vi "ArrayBuffer_main.vi"() -> ()   [LabVIEW 2020]
uses:
  <vilib>/numeric/Random Number (Range) U64.vi
  <vilib>/numeric/sub_Random U32.vi
  Desktop/AddrToValue.dll
  Desktop/Dll_Lib_DAQ_Child.dll
  Desktop/Dll_Lib_DAQ.dll
panel:
  out "First Run Com?":bool
  out "initialized array 2":i32[](array[numeric])
  out "initialized array":i32[](array[numeric])
  out "DBL 2":dbl
  out "string 2":string
  out "Array":i32[](array[numeric])
  out "string":string
  out "error out":errorcluster
  out "DBL":dbl
  in  "input":T1={"DBL"=10.0, "String (50 Character Limit)"="abcd", "Array (50 Element Limit)"=[10, 100]}
  out "output array":i32[](array[numeric])
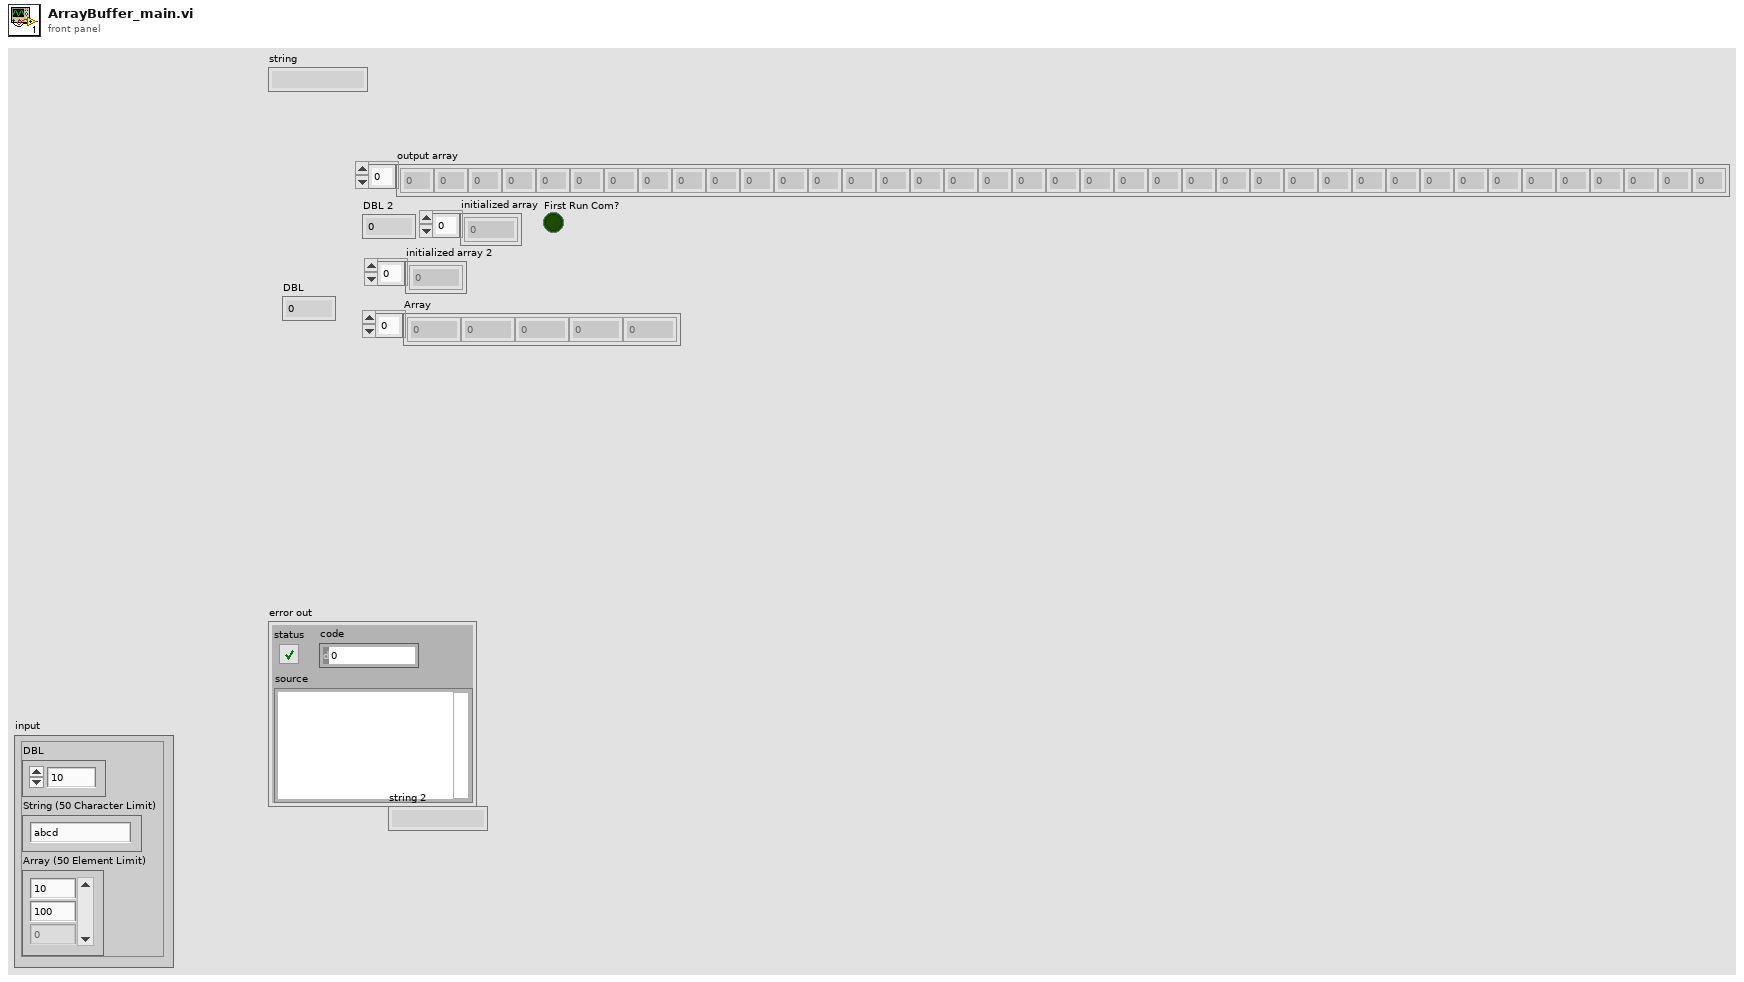
[diagram p1: front panel]
types:
  T1 = cluster{"DBL":dbl, "String (50 Character Limit)":string, "Array (50 Element Limit)":i32[]}
  T2 = cluster{"unsigned byte array[0]":u8, "unsigned byte array[1]":u8, "unsigned byte array[2]":u8, "unsigned byte array[3]":u8, "unsigned byte array[4]":u8, "unsigned byte array[5]":u8, "unsigned byte array[6]":u8, "unsigned byte array[7]":u8, "unsigned byte array[8]":u8, "unsigned byte array[9]":u8, "unsigned byte array[10]":u8, "unsigned byte array[11]":u8, "unsigned byte array[12]":u8, "unsigned byte array[13]":u8, "unsigned byte array[14]":u8, "unsigned byte array[15]":u8, "unsigned byte array[16]":u8, "unsigned byte array[17]":u8, "unsigned byte array[18]":u8, "unsigned byte array[19]":u8, "unsigned byte array[20]":u8, "unsigned byte array[21]":u8, "unsigned byte array[22]":u8, "unsigned byte array[23]":u8, "unsigned byte array[24]":u8, "unsigned byte array[25]":u8, "unsigned byte array[26]":u8, "unsigned byte array[27]":u8, "unsigned byte array[28]":u8, "unsigned byte array[29]":u8, "unsigned byte array[30]":u8, "unsigned byte array[31]":u8, "unsigned byte array[32]":u8, "unsigned byte array[33]":u8, "unsigned byte array[34]":u8, "unsigned byte array[35]":u8, "unsigned byte array[36]":u8, "unsigned byte array[37]":u8, "unsigned byte array[38]":u8, "unsigned byte array[39]":u8, "unsigned byte array[40]":u8, "unsigned byte array[41]":u8, "unsigned byte array[42]":u8, "unsigned byte array[43]":u8, "unsigned byte array[44]":u8, "unsigned byte array[45]":u8, "unsigned byte array[46]":u8, "unsigned byte array[47]":u8, "unsigned byte array[48]":u8, "unsigned byte array[49]":u8, "unsigned byte array[50]":u8}
  T3 = cluster{"DBL":dbl, "unsigned byte array":cluster{"unsigned byte array[0]":u8, "unsigned byte array[1]":u8, "unsigned byte array[2]":u8, "unsigned byte array[3]":u8, "unsigned byte array[4]":u8, "unsigned byte array[5]":u8, "unsigned byte array[6]":u8, "unsigned byte array[7]":u8, "unsigned byte array[8]":u8, "unsigned byte array[9]":u8, "unsigned byte array[10]":u8, "unsigned byte array[11]":u8, "unsigned byte array[12]":u8, "unsigned byte array[13]":u8, "unsigned byte array[14]":u8, "unsigned byte array[15]":u8, "unsigned byte array[16]":u8, "unsigned byte array[17]":u8, "unsigned byte array[18]":u8, "unsigned byte array[19]":u8, "unsigned byte array[20]":u8, "unsigned byte array[21]":u8, "unsigned byte array[22]":u8, "unsigned byte array[23]":u8, "unsigned byte array[24]":u8, "unsigned byte array[25]":u8, "unsigned byte array[26]":u8, "unsigned byte array[27]":u8, "unsigned byte array[28]":u8, "unsigned byte array[29]":u8, "unsigned byte array[30]":u8, "unsigned byte array[31]":u8, "unsigned byte array[32]":u8, "unsigned byte array[33]":u8, "unsigned byte array[34]":u8, "unsigned byte array[35]":u8, "unsigned byte array[36]":u8, "unsigned byte array[37]":u8, "unsigned byte array[38]":u8, "unsigned byte array[39]":u8, "unsigned byte array[40]":u8, "unsigned byte array[41]":u8, "unsigned byte array[42]":u8, "unsigned byte array[43]":u8, "unsigned byte array[44]":u8, "unsigned byte array[45]":u8, "unsigned byte array[46]":u8, "unsigned byte array[47]":u8, "unsigned byte array[48]":u8, "unsigned byte array[49]":u8, "unsigned byte array[50]":u8}, i32[]}
  T4 = cluster{"DBL":dbl, "unsigned byte array":cluster{"unsigned byte array[0]":u8, "unsigned byte array[1]":u8, "unsigned byte array[2]":u8, "unsigned byte array[3]":u8, "unsigned byte array[4]":u8, "unsigned byte array[5]":u8, "unsigned byte array[6]":u8, "unsigned byte array[7]":u8, "unsigned byte array[8]":u8, "unsigned byte array[9]":u8, "unsigned byte array[10]":u8, "unsigned byte array[11]":u8, "unsigned byte array[12]":u8, "unsigned byte array[13]":u8, "unsigned byte array[14]":u8, "unsigned byte array[15]":u8, "unsigned byte array[16]":u8, "unsigned byte array[17]":u8, "unsigned byte array[18]":u8, "unsigned byte array[19]":u8, "unsigned byte array[20]":u8, "unsigned byte array[21]":u8, "unsigned byte array[22]":u8, "unsigned byte array[23]":u8, "unsigned byte array[24]":u8, "unsigned byte array[25]":u8, "unsigned byte array[26]":u8, "unsigned byte array[27]":u8, "unsigned byte array[28]":u8, "unsigned byte array[29]":u8, "unsigned byte array[30]":u8, "unsigned byte array[31]":u8, "unsigned byte array[32]":u8, "unsigned byte array[33]":u8, "unsigned byte array[34]":u8, "unsigned byte array[35]":u8, "unsigned byte array[36]":u8, "unsigned byte array[37]":u8, "unsigned byte array[38]":u8, "unsigned byte array[39]":u8, "unsigned byte array[40]":u8, "unsigned byte array[41]":u8, "unsigned byte array[42]":u8, "unsigned byte array[43]":u8, "unsigned byte array[44]":u8, "unsigned byte array[45]":u8, "unsigned byte array[46]":u8, "unsigned byte array[47]":u8, "unsigned byte array[48]":u8, "unsigned byte array[49]":u8, "unsigned byte array[50]":u8}, "unsigned byte array":cluster{"unsigned byte array[0]":u8, "unsigned byte array[1]":u8, "unsigned byte array[2]":u8, "unsigned byte array[3]":u8, "unsigned byte array[4]":u8, "unsigned byte array[5]":u8, "unsigned byte array[6]":u8, "unsigned byte array[7]":u8, "unsigned byte array[8]":u8, "unsigned byte array[9]":u8, "unsigned byte array[10]":u8, "unsigned byte array[11]":u8, "unsigned byte array[12]":u8, "unsigned byte array[13]":u8, "unsigned byte array[14]":u8, "unsigned byte array[15]":u8, "unsigned byte array[16]":u8, "unsigned byte array[17]":u8, "unsigned byte array[18]":u8, "unsigned byte array[19]":u8, "unsigned byte array[20]":u8, "unsigned byte array[21]":u8, "unsigned byte array[22]":u8, "unsigned byte array[23]":u8, "unsigned byte array[24]":u8, "unsigned byte array[25]":u8, "unsigned byte array[26]":u8, "unsigned byte array[27]":u8, "unsigned byte array[28]":u8, "unsigned byte array[29]":u8, "unsigned byte array[30]":u8, "unsigned byte array[31]":u8, "unsigned byte array[32]":u8, "unsigned byte array[33]":u8, "unsigned byte array[34]":u8, "unsigned byte array[35]":u8, "unsigned byte array[36]":u8, "unsigned byte array[37]":u8, "unsigned byte array[38]":u8, "unsigned byte array[39]":u8, "unsigned byte array[40]":u8, "unsigned byte array[41]":u8, "unsigned byte array[42]":u8, "unsigned byte array[43]":u8, "unsigned byte array[44]":u8, "unsigned byte array[45]":u8, "unsigned byte array[46]":u8, "unsigned byte array[47]":u8, "unsigned byte array[48]":u8, "unsigned byte array[49]":u8, "unsigned byte array[50]":u8}}
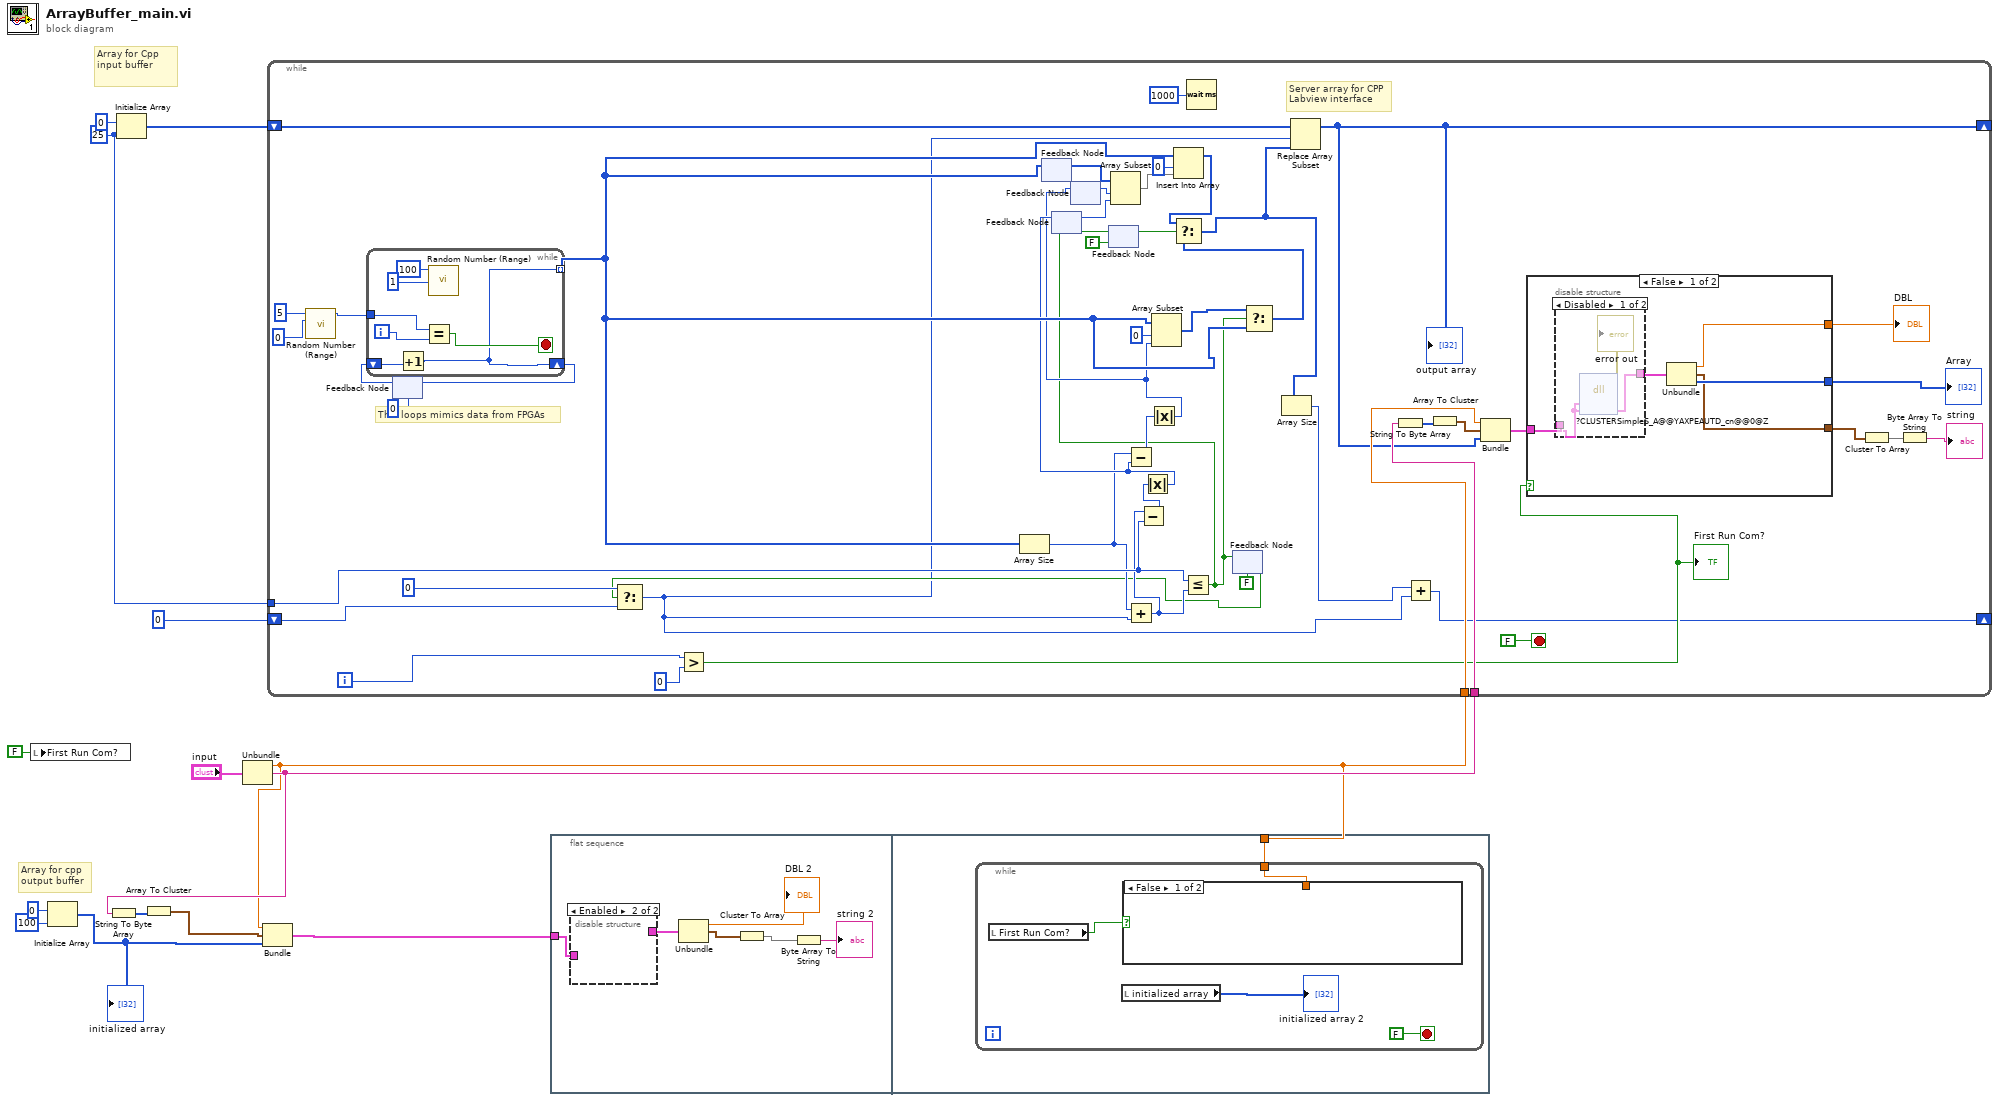
[diagram p0: block diagram]
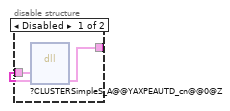
[diagram p2: hidden frame]
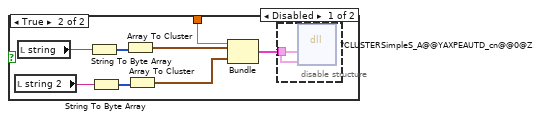
[diagram p3: hidden frame]
diagram:
  w11 = 25 ("dimension size")
  # "Array for cpp \noutput buffer"
  # "Array for Cpp \ninput buffer"
  n1 = local write "First Run Com?"(FALSE ("First Run Com?")) -> ()
  n2 = Initialize Array(0 ("element"), 100 ("dimension size")) -> (w7:i32[])
  "initialized array" <- w7
  n3 = Initialize Array(0 ("element"), w11) -> (w13:i32[])
  n4 = Unbundle("input") -> ("DBL"=w2:dbl, "String (50 Character Limit)"=w5:string)  [unwired: 1 out]
  n5 = String To Byte Array(string=w5) -> (unsigned byte array=w6:u8[])
  n6 = Array To Cluster(array=w6) -> (cluster=w4:T2)
  n7 = Bundle("DBL"=w2, "unsigned byte array"=w4, w7) -> (w3:T3)  [unwired: 1 out]
  n8 = while {
    shift-right: [w51] -> _
    shift-left: w13 -> [w64]
    shift-right: [w19] -> _
    shift-left: 0 -> [w21]
    tunnel: w11 -> [w43]
    tunnel: w2 -> [w54]
    tunnel: w5 -> [w56]
    i -> [w17]
    stop <- FALSE stop-if-true
    # "This loops mimics data from FPGAs"
    # "Server array for CPP\nLabview interface"
    n9 = call-poly <vilib>:"Random Number (Range).vi"("lower bound (0)"=u64 0, "upper bound (100)"=u64 5) -> ("number"=w15:u64)  [unwired: 9 in]
    n10 = feedback #1(0) -> (w61:i32)
    n11 = while {
      tunnel: w15 -> [w76]
      tunnel: [w74] -> w31 mode=indexing
      shift-right: [w74] -> w59
      shift-left: w61 -> [w77]
      i -> [w75]
      stop <- w80 stop-if-true
      n12 = Increment(x=w77) -> (x+1=w74:i32)
      n13 = Equal?(x=w76, y=w75) -> (x = y?=w80:bool)
      n14 = call-poly <vilib>:"Random Number (Range).vi"("lower bound (0)"=u64 1, "upper bound (100)"=u64 100) -> ()  [unwired: 9 in, 1 out]
    }
    n15 = feedback-in #1(w59) -> ()
    n16 = Greater?(x=w17, y=0 ("x")) -> (0:w47:bool)
    "First Run Com?" <- w47
    n17 = Array Size(array=w31) -> (size(s)=w23:i32)
    n18 = feedback #2() -> (w30:i32[])  [unwired: 1 in]
    n19 = feedback-in #2(w31) -> ()
    n20 = feedback #3() -> (w27:i32)  [unwired: 1 in]
    n21 = feedback #4() -> (w29:i32)  [unwired: 1 in]
    n22 = feedback #5(FALSE) -> (w40:bool)
    n23 = Array Subset(array=w30, index=w29, length=w27) -> (w38:i32[])
    n24 = Insert Into Array(array=w31, index=0, new element=w38) -> (w36:i32[])
    n25 = Wait (ms)(milliseconds to wait=u32 1000) -> ()  [unwired: 1 out]
    n26 = feedback #6(FALSE) -> (w22:bool)
    n27 = Select(t=0, s=w22, f=w21) -> (s? t:f=w18:i32)
    n28 = Add(x=w23, y=w18) -> (x+y=w24:i32)
    n29 = Subtract(x=w24, y=w43) -> (x-y=w32:i32)
    n30 = Absolute Value(x=w32) -> (abs(x)=w28:i32)
    n31 = feedback-in #3(w28) -> ()
    n32 = Subtract(x=w23, y=w28) -> (x-y=w33:i32)
    n33 = Absolute Value(x=w33) -> (abs(x)=w26:i32)
    n34 = feedback-in #4(w26) -> ()
    n35 = Array Subset(array=w31, index=0, length=w26) -> (w42:i32[])
    n36 = Less Or Equal?(x=w43, y=w24) -> (x <= y?=w25:bool)
    n37 = feedback-in #5(w25) -> ()
    n38 = feedback-in #6(w25) -> ()
    n39 = Select(t=w42, s=w25, f=w31) -> (s? t:f=w39:i32[])
    n40 = Select(t=w36, s=w40, f=w39) -> (s? t:f=w35:i32[])
    n41 = Array Size(array=w35) -> (size(s)=w20:i32)
    n42 = Replace Array Subset(array=w64, new element=w35, index=w18) -> (w51:i32[])
    "output array" <- w51
    n43 = String To Byte Array(string=w56) -> (unsigned byte array=w55:u8[])
    n44 = Add(x=w20, y=w18) -> (x+y=w19:i32)
    n45 = Array To Cluster(array=w55) -> (cluster=w53:T2)
    n46 = Bundle("DBL"=w54, "unsigned byte array"=w53, w51) -> (w52:T3)  [unwired: 1 out]
    n47 = case shown="False" w47 {
      tunnel: w52 -> [w70 _]
      tunnel: [w68 _] -> w49
      tunnel: [w67 _] -> w48
      tunnel: [w66 _] -> w46
      frame False {
        n48 = disable-structure shown="Disabled" {
          disable-tunnel: w70 -> [w73 _]
          disable-tunnel: [w72 _] -> w69
          frame Disabled {
            n49 = dll-call lib="C:/Users/Himal/Desktop/Dll_Lib_DAQ.dll" fn="?CLUSTERSimpleS_A@@YAXPEAUTD_cn@@0@Z"("input"=w73, "output"=w73) -> (error out=→"error out":errorcluster, "output"=w72:T3)  [unwired: 5 in, 1 out]
          }
          frame Enabled {
          }
        }
        n50 = Unbundle(w69) -> ("DBL"=w67:dbl, "unsigned byte array"=w66:T2, w68:i32[])
      }
      frame True {
      }
    }
    "DBL" <- w48
    "Array" <- w49
    n51 = Cluster To Array(cluster=w46) -> (array=w45:u8[])
    n52 = Byte Array To String(unsigned byte array=w45) -> (string=→"string":string)
  }
  n53 = flat-sequence {
    tunnel: w3 -> [w81]
    tunnel: w2 -> [w89]
    frame #0 {
      n54 = disable-structure shown="Enabled" {
        disable-tunnel: [w88 _] -> w82
        disable-tunnel: w81 -> [w87 _]
        frame Disabled {
          n55 = dll-call lib="C:/Users/Himal/Desktop/Dll_Lib_DAQ_Child.dll" fn="?CLUSTERSimpleS_A@@YAXPEAUTD_cn@@0@Z"("input"=w87, "output"=w87) -> ("output"=w88:T3)  [unwired: 5 in, 2 out]
        }
        frame Enabled {
        }
      }
      n56 = Unbundle(w82) -> ("DBL"=→"DBL 2":dbl, "unsigned byte array"=w85:T2)  [unwired: 1 out]
      n57 = Cluster To Array(cluster=w85) -> (array=w83:u8[])
      n58 = Byte Array To String(unsigned byte array=w83) -> (string=→"string 2":string)
    }
    frame #1 {
      n59 = while {
        tunnel: w89 -> [w93]
        stop <- FALSE stop-if-true
        n60 = local read "First Run Com?"() -> (w90:bool)
        n61 = local read "initialized array"() -> (→"initialized array 2":i32[])
        n62 = case shown="False" w90 {
          tunnel: w93 -> [_ w95]
          frame False {
          }
          frame True {
            n63 = local read "string 2"() -> (w99:string)
            n64 = local read "string"() -> (w97:string)
            n65 = String To Byte Array(string=w97) -> (unsigned byte array=w96:u8[])
            n66 = String To Byte Array(string=w99) -> (unsigned byte array=w98:u8[])
            n67 = Array To Cluster(array=w96) -> (cluster=w100:T2)
            n68 = Array To Cluster(array=w98) -> (cluster=w101:T2)
            n69 = Bundle("DBL"=w95, "unsigned byte array"=w100, "unsigned byte array"=w101) -> (w94:T4)  [unwired: 1 out]
            n70 = disable-structure shown="Disabled" {
              disable-tunnel: w94 -> [w102 _]
              frame Disabled {
                n71 = dll-call lib="C:/Users/Himal/Desktop/AddrToValue.dll" fn="?CLUSTERSimpleS_A@@YAXPEAUTD_cn@@0@Z"("input"=w102, "output"=w102) -> ()  [unwired: 6 in, 2 out]
              }
              frame Enabled {
              }
            }
          }
        }
      }
    }
  }
